vi "Receive Data Batch.vi"(8 "Error in":errorcluster, 11 "State Variables in":T1={"Stop Notifier"=refnum, "UI References"=[], "DAQmx"={"ECG Input"={"Channel"="", "Task"="", "Max Value"=0.0, "Min Value"=0.0, "Sampling Rate"=0.0, "Batch Size"=10}, "Trigger Output"={"Channel"="", "Task"="", "Pulse Frequency"=0.0, "Delay"=0, "Triggers per Shot"=0}}, "Data Queue"=refnum, "Filter"={"Batch Size"=1000, "Update Cycle"=0, "Filter Buffer"=[]}, "Last Detect Result"=FALSE}) -> (0 "Error out":errorcluster, 2 "Buffered Data":dbl[](array[numeric]), 3 "State Variables out":T1={"Stop Notifier"=refnum, "UI References"=[], "DAQmx"={"ECG Input"={"Channel"="", "Task"="", "Max Value"=0.0, "Min Value"=0.0, "Sampling Rate"=0.0, "Batch Size"=10}, "Trigger Output"={"Channel"="", "Task"="", "Pulse Frequency"=0.0, "Delay"=0, "Triggers per Shot"=0}}, "Data Queue"=refnum, "Filter"={"Batch Size"=1000, "Update Cycle"=0, "Filter Buffer"=[]}, "Last Detect Result"=FALSE}, 5 "Ready?":bool)   [LabVIEW 2014, in "Filter.lvlib"]
uses:
  Filter.lvlib
  Controls/State Variables.ctl
  Controls/DAQmx Variables.ctl
  Controls/Filter Variables.ctl
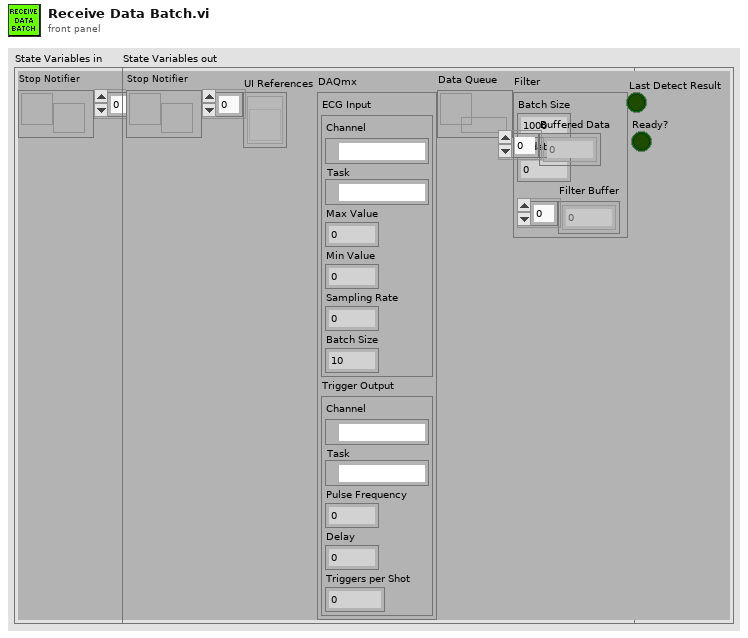
[diagram p1: front panel]
types:
  T1 = typedef "State Variables.ctl" = cluster{"Stop Notifier":refnum<notifier>, "UI References":refnum<vi>[], "DAQmx":T2, "Data Queue":refnum<queue>, "Filter":T3, "Last Detect Result":bool}
  T2 = typedef "DAQmx Variables.ctl" = cluster{"ECG Input":cluster{"Channel":tag, "Task":refnum<k21>, "Max Value":dbl, "Min Value":dbl, "Sampling Rate":dbl, "Batch Size":i32}, "Trigger Output":cluster{"Channel":tag, "Task":refnum<k21>, "Pulse Frequency":dbl, "Delay":u16, "Triggers per Shot":i32}}
  T3 = typedef "Filter Variables.ctl" = cluster{"Batch Size":i32, "Update Cycle":i32, "Filter Buffer":dbl[]}
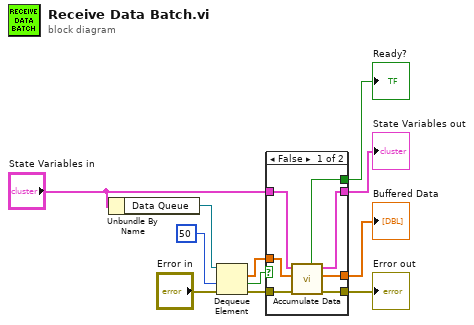
[diagram p0: block diagram]
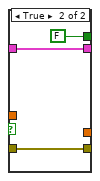
[diagram p2: hidden frame]
diagram:
  n1 = Unbundle By Name("State Variables in") -> ("Data Queue"=w10:refnum<queue>)
  n2 = Dequeue Element(queue=w10, timeout in ms (-1)=50, error in (no error)="Error in") -> (element=w1:dbl[], timed out?=w2:bool, error out=w3:errorcluster)  [unwired: 1 out]
  n3 = case shown="False" w2 {
    tunnel: "State Variables in" -> [w18 w20]
    tunnel: [w17 w20] -> w7
    tunnel: [w16 FALSE ("Is Buffer Ready?")] -> w6
    tunnel: [w15 _] -> w5
    tunnel: [w14 w21] -> w4
    tunnel: w3 -> [w13 w21]
    tunnel: w1 -> [w12 _]
    frame False {
      n4 = call "Accumulate Data.vi"("Error in"=w13, "New Data"=w12, "State Variables in"=w18) -> ("Error out"=w14:errorcluster, "Buffered Data"=w15:dbl[], "State Variables out"=w17:T1, "Is Buffer Ready?"=w16:bool)  [unwired: 5 in]
    }
    frame True {
    }
  }
  "Error out" <- w4
  "State Variables out" <- w7
  "Buffered Data" <- w5
  "Ready?" <- w6
